vi "FG Left Velocity.vi"(2 "FG Action (Read)":T1, 3 "Left Velocity In (RPM)":dbl) -> (1 "Left Velocity Out (RPM)":dbl)   [LabVIEW 2009]
uses:
  Actions for FG's.ctl
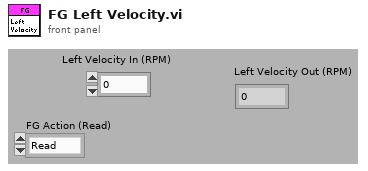
[diagram p1: front panel]
types:
  T1 = typedef "Actions for FG's.ctl" = enum16{"Read", "Write"}
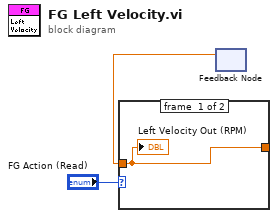
[diagram p0: block diagram]
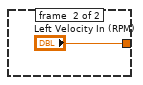
[diagram p2: hidden frame]
diagram:
  n1 = feedback #1() -> (w1:dbl)  [unwired: 1 in]
  n2 = case shown="\"Write\"" "FG Action (Read)" {
    tunnel: [w4 "Left Velocity In (RPM)"] -> w2
    tunnel: w1 -> [w4 _]
    frame #0 {
      "Left Velocity Out (RPM)" <- w4
    }
    frame #1 {
    }
  }
